vi "maze_v10.vi"   [LabVIEW 2012]
uses:
  <vilib>/NXT/Subs/MotorOutput.ctl
  <vilib>/NXT/Block Support/NXT_InputPort.ctl
  <vilib>/NXT/Dual Mode Library/prims/addArrayElements_int.vi
  <vilib>/NXT/Dual Mode Library/Waits/Wait_Num(msec).vi
  <vilib>/NXT/Dual Mode Library/Sound/Tone.vi
types:
  T1 = typedef "MotorOutput.ctl" = u8
  T2 = typedef "LVHSConnector.ctl" = cluster{"Hardware":string, "Flattened String":string}
  T3 = typedef "NXT_InputPort.ctl" = u8
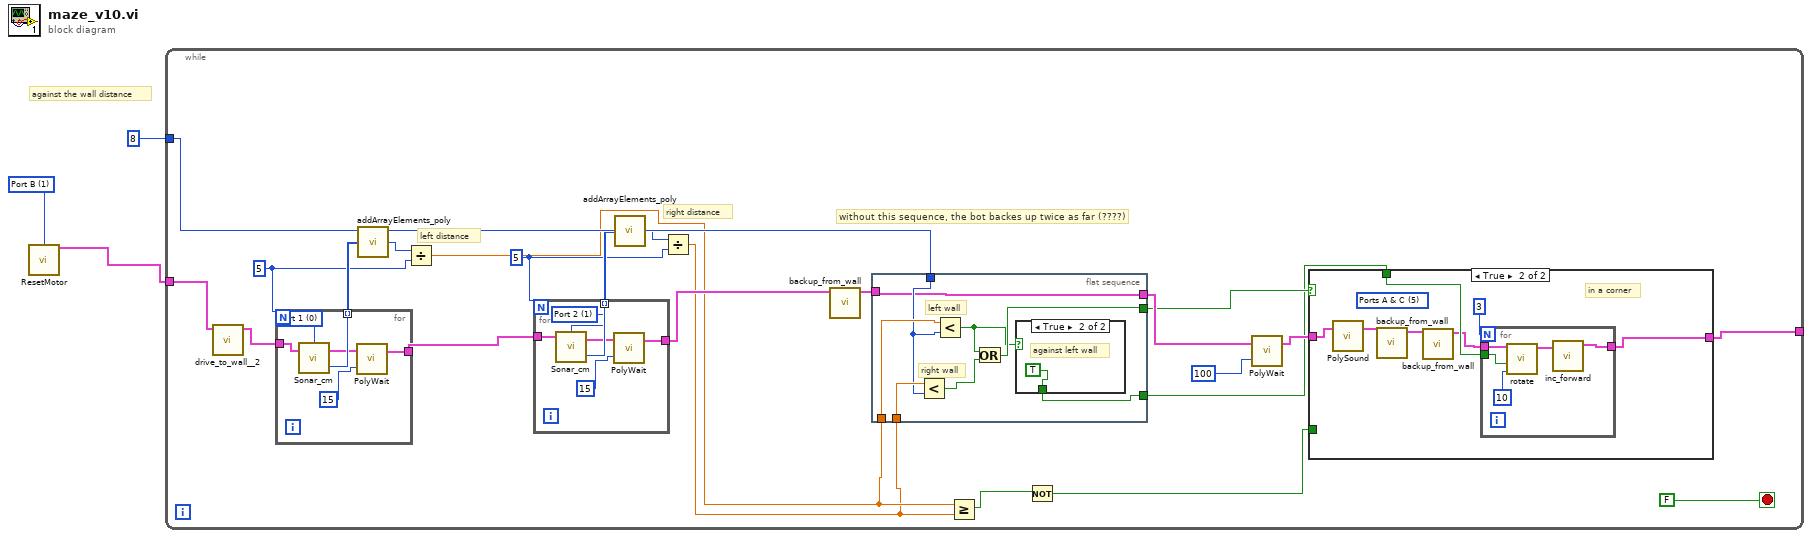
[diagram p0: block diagram]
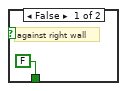
[diagram p2: hidden frame]
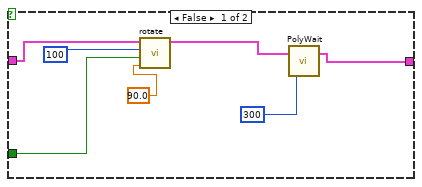
[diagram p3: hidden frame]
diagram:
  w3 = T1 1 items=["Port A"=0, "Port B"=1, "Port C"=2, "Ports A & B"=4, "Ports A & C"=5, "Ports B & C"=6, "All Ports"=3] ("Output Port (All Ports)")
  # "against the wall distance"
  n1 = call <vilib>:"ResetMotor.vi"("Port (All Ports)"=w3) -> ("NXT"=w1:T2)  [unwired: 3 in]
  n2 = while {
    tunnel: u16 8 ("power") -> [w21]
    tunnel: [w4] -> _
    tunnel: w1 -> [w6]
    stop <- FALSE stop-if-true
    w12 = 5
    w15 = 5
    # "right distance"
    # "left distance"
    # "without this sequence, the bot backes up twice as far (????)"
    n3 = call "drive_to_wall__2.vi"("NXT"=w6) -> ("NXT 2"=w5:T2)  [unwired: 10 in]
    n4 = for {
      N: w15 -> [_]
      tunnel: [w38] -> w17 mode=indexing
      tunnel: [w36] -> w11
      tunnel: w5 -> [w33]
      w34 = T3 0 items=["Port 1", "Port 2", "Port 3", "Port 4"] ("Port (Port 4)")
      n5 = call <vilib>:"Sonar_cm.vi"("NXT"=w33, "Port (Port 4)"=w34) -> ("Distance (cm)"=w38:i16, "NXT"=w37:T2)  [unwired: 1 in]
      n6 = call-poly <vilib>:"PolyWait.vi"("Time (100 msec)"=15, "NXT"=w37) -> ("NXT"=w36:T2)  [unwired: 2 in]
    }
    n7 = call-poly <vilib>:"addArrayElements_poly.vi"("Numeric Array"=w17) -> ("Sum"=w16:i32)
    n8 = Divide(x=w16, y=w15) -> (x/y=w8:dbl)
    n9 = for {
      N: w12 -> [_]
      tunnel: w11 -> [w31]
      tunnel: [w32] -> w14 mode=indexing
      tunnel: [w29] -> w10
      w27 = T3 1 items=["Port 1", "Port 2", "Port 3", "Port 4"] ("Port (Port 4)")
      n10 = call <vilib>:"Sonar_cm.vi"("NXT"=w31, "Port (Port 4)"=w27) -> ("Distance (cm)"=w32:i16, "NXT"=w30:T2)  [unwired: 1 in]
      n11 = call-poly <vilib>:"PolyWait.vi"("Time (100 msec)"=15, "NXT"=w30) -> ("NXT"=w29:T2)  [unwired: 2 in]
    }
    n12 = call-poly <vilib>:"addArrayElements_poly.vi"("Numeric Array"=w14) -> ("Sum"=w13:i32)
    n13 = Divide(x=w13, y=w12) -> (x/y=w7:dbl)
    n14 = call "backup_from_wall.vi"("NXT"=w10) -> ("NXT2"=w18:T2)  [unwired: 10 in]
    n15 = flat-sequence {
      tunnel: [w39] -> w24
      tunnel: w7 -> [w46]
      tunnel: w21 -> [w44]
      tunnel: w8 -> [w45]
      tunnel: [w42] -> w20
      tunnel: [w40] -> w19
      tunnel: w18 -> [w39]
      frame #0 {
        # "left wall"
        # "right wall"
        n16 = Less?(x=w46, y=w44) -> (x < y?=w43:bool)
        n17 = Less?(x=w45, y=w44) -> (x < y?=w41:bool)
        n18 = Or(x=w41, y=w43) -> (x .or. y?=w42:bool)
        n19 = case shown="True" w41 {
          tunnel: [FALSE TRUE] -> w40
          frame False {
            # "against right wall"
          }
          frame True {
            # "against left wall"
          }
        }
      }
    }
    n20 = Greater Or Equal?(x=w8, y=w7) -> (x >= y?=w9:bool)
    n21 = Not(x=w9) -> (.not. x?=w25:bool)
    n22 = call-poly <vilib>:"PolyWait.vi"("Time (100 msec)"=u16 100 ("power"), "NXT"=w24) -> ("NXT"=w23:T2)  [unwired: 2 in]
    n23 = case shown="True" w20 {
      tunnel: w19 -> [_ w59]
      tunnel: w23 -> [w50 w56]
      tunnel: [w49 w57] -> w4
      tunnel: w25 -> [w53 _]
      frame False {
        n24 = call "rotate.vi"("degrees to  rotate"=90.0, "right(T)/left(F)"=w53, "power"=u16 100, "NXT 2"=w50) -> ("NXT"=w55:T2)  [unwired: 7 in]
        n25 = call-poly <vilib>:"PolyWait.vi"("Time (100 msec)"=i16 300 ("degrees to  rotate"), "NXT"=w55) -> ("NXT"=w49:T2)  [unwired: 2 in]
      }
      frame True {
        (unwired) T1 5 items=["Port A"=0, "Port B"=1, "Port C"=2, "Ports A & B"=4, "Ports A & C"=5, "Ports B & C"=6, "All Ports"=3] ("Output Port (All Ports)")
        # "in a corner"
        n26 = call-poly <vilib>:"PolySound.vi"("NXT"=w56) -> ("NXT"=w62:T2)  [unwired: 3 in]
        n27 = call "backup_from_wall.vi"("NXT"=w62) -> ("NXT2"=w61:T2)  [unwired: 10 in]
        n28 = call "backup_from_wall.vi"("NXT"=w61) -> ("NXT2"=w58:T2)  [unwired: 10 in]
        n29 = for {
          N: u16 3 ("power") -> [_]
          tunnel: w59 -> [w66]
          tunnel: w58 -> [w65]
          tunnel: [w63] -> w57
          n30 = call "rotate.vi"("degrees to  rotate"=u16 10 ("power"), "right(T)/left(F)"=w66, "NXT 2"=w65) -> ("NXT"=w64:T2)  [unwired: 8 in]
          n31 = call "inc_forward.vi"("NXT"=w64) -> ("NXT2"=w63:T2)  [unwired: 10 in]
        }
      }
    }
  }
